vi "Finish.vi"   [LabVIEW 2017]
doc: "This VI is called just before exiting. It is expected to close I/O refnum, save collected data, etc."
uses:
  <vilib>/Rock Robotics/WPI/Utilities/WPI_GetSetVariantRefNum.vi
types:
  T1 = typedef "WPI_CompressorDevRef.ctl" = cluster{"DevStatus":errorcluster, "Pneumatics Control Module":u8}
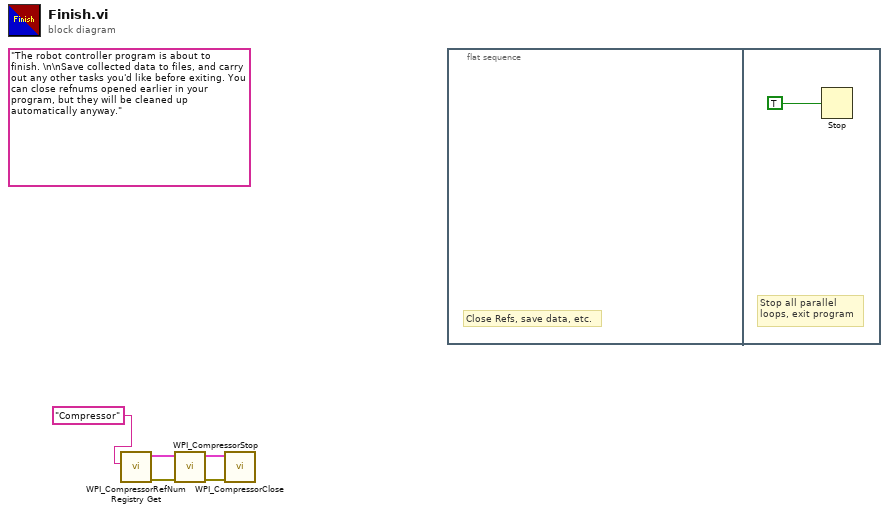
[diagram p0: block diagram]
diagram:
  (unwired) "The robot controller program is about to finish. \n\nSave collected data to files, and carry out any other tasks you'd like before exiting. You can close refnums opened earlier in your program, but they will be cleaned up automatically anyway."
  n1 = call <vilib>:"WPI_CompressorRefNum Registry Get.vi"("refnum name"="Compressor") -> ("error out"=w5:errorcluster, "CompressorDevRef"=w4:T1)  [unwired: 9 in]
  n2 = call <vilib>:"WPI_CompressorStop.vi"("error in (no error)"=w5, "CompressorDevRef"=w4) -> ("error out"=w3:errorcluster, "CompressorDevRef"=w2:T1)  [unwired: 8 in]
  n3 = call <vilib>:"WPI_CompressorClose.vi"("error in (no error)"=w3, "CompressorDevRef"=w2) -> ()  [unwired: 9 in, 1 out]
  n4 = flat-sequence {
    frame #0 {
      # "Close Refs, save data, etc."
    }
    frame #1 {
      # "Stop all parallel\nloops, exit program"
      n5 = Stop(stop? (T)=TRUE ("Quit")) -> ()
    }
  }
